vi "Panel Registry.vi"(8 "error in (no error)":errorcluster) -> (0 "error out":errorcluster, 3 "Panel Registry out":refnum<class "Panel Registry.lvclass">)   [LabVIEW 2017, in "MGI-Panel Manager.lvlib" / "Panel Registry.lvclass"]
doc: "Creates a Panel Registry.\n\n----\nPlease see the following web address for additional documentation and tutorial information:\nhttp://www.mooregoodideas.com/mgi-panel-manager/\n\nAuthor: Derek Trepanier\n\nCopyright (c) 2018, Moore Good Ideas, Inc.\n\nAll rights reserved.\n\nRedistribution and use in source and binary forms, with or without modification, are permitted provided that the following conditions are met:\n\n * Redistributions of source code must retain the above copyright notice, this list of conditions and the following disclaimer.\n * Redistributions in binary form must reproduce the above copyright notice, this list of conditions and the following disclaimer in the documentation and/or other materials provided with the distribution.\n * Neither the name of Moore Good Ideas, Inc. nor the names of its contributors may be used to endorse or promote products derived from this software without specific prior written permission.\n\nTHIS SOFTWARE IS PROVIDED BY THE COPYRIGHT HOLDERS AND CONTRIBUTORS \"AS IS\" AND ANY EXPRESS OR IMPLIED WARRANTIES, INCLUDING, BUT NOT LIMITED TO, THE IMPLIED WARRANTIES OF MERCHANTABILITY AND FITNESS FOR A PARTICULAR PURPOSE ARE DISCLAIMED. IN NO EVENT SHALL THE COPYRIGHT OWNER OR CONTRIBUTORS BE LIABLE FOR ANY DIRECT, INDIRECT, INCIDENTAL, SPECIAL, EXEMPLARY, OR CONSEQUENTIAL DAMAGES (INCLUDING, BUT NOT LIMITED TO, PROCUREMENT OF SUBSTITUTE GOODS OR SERVICES; LOSS OF USE, DATA, OR PROFITS; OR BUSINESS INTERRUPTION) HOWEVER CAUSED AND ON ANY THEORY OF LIABILITY, WHETHER IN CONTRACT, STRICT LIABILITY, OR TORT (INCLUDING NEGLIGENCE OR OTHERWISE) ARISING IN ANY WAY OUT OF THE USE OF THIS SOFTWARE, EVEN IF ADVISED OF THE POSSIBILITY OF SUCH DAMAGE."
uses:
  Panel Registry.lvclass
  Panel Registry.lvclass/Panel Registry.ctl
  Static.vi
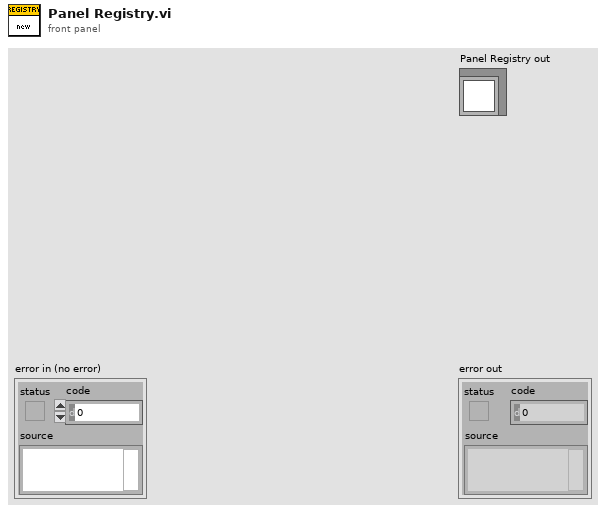
[diagram p1: front panel]
types:
  T1 = typedef "Semaphore RefNum" = refnum<k1>
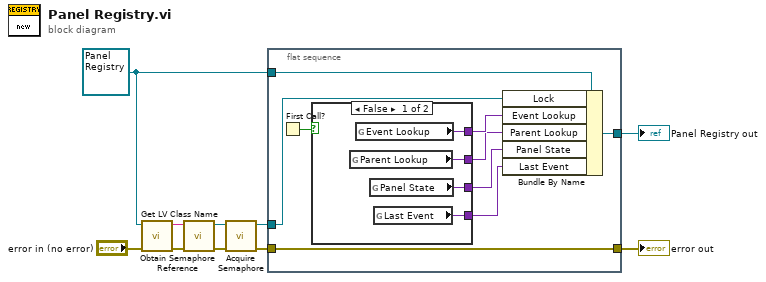
[diagram p0: block diagram]
diagram:
  w10 = refnum<class "Panel Registry.lvclass"> refnum ("Panel Registry in")
  n1 = call <vilib>:"Get LV Class Name.vi"("error in (no error)"="error in (no error)", "object"=w10) -> ("error out"=w6:errorcluster, "class name"=w9:string)  [unwired: 8 in]
  n2 = call <vilib>:"Obtain Semaphore Reference.vi"("error in (no error)"=w6, "name (unnamed)"=w9) -> ("error out"=w5:errorcluster, "semaphore"=w4:T1)  [unwired: 3 in, 1 out]
  n3 = call <vilib>:"Acquire Semaphore.vi"("error in (no error)"=w5, "semaphore"=w4) -> ("error out"=w1:errorcluster, "semaphore out"=w3:T1)  [unwired: 3 in, 1 out]
  n4 = flat-sequence {
    tunnel: w10 -> [w19]
    tunnel: [w18] -> w8
    tunnel: w3 -> [w17]
    tunnel: [w14] -> w2
    tunnel: w1 -> [w14]
    frame #0 {
      n5 = First Call?() -> (First Call?: T/F=w13:bool)
      n6 = case shown="False" w13 {
        tunnel: [w23 _] -> w16
        tunnel: [w22 _] -> w15
        tunnel: [w21 _] -> w12
        tunnel: [w20 _] -> w11
        frame False {
          n7 = global read "Static.vi" "Parent Lookup"() -> (w22:variant)
          n8 = global read "Static.vi" "Event Lookup"() -> (w23:variant)
          n9 = global read "Static.vi" "Panel State"() -> (w21:variant)
          n10 = global read "Static.vi" "Last Event"() -> (w20:variant)
        }
        frame True {
        }
      }
      n11 = Bundle By Name(cluster=w19, "Lock"=w17, "Event Lookup"=w16, "Parent Lookup"=w15, "Panel State"=w12, "Last Event"=w11) -> (w18:refnum<class "Panel Registry.lvclass">)
    }
  }
  "error out" <- w2
  "Panel Registry out" <- w8
